vi "Parse Sonar Data.vi"(1 "Sonar Values String":string) -> (0 "Sonar Data":i32[](array[numeric]))   [LabVIEW 2020, in "Advent of Code.lvlib"]
uses:
  Advent of Code.lvlib
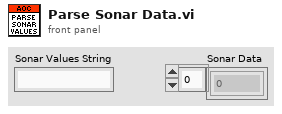
[diagram p1: front panel]
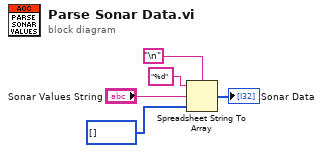
[diagram p0: block diagram]
diagram:
  n1 = Spreadsheet String To Array(delimiter (Tab)="\n", format string="%d", spreadsheet string="Sonar Values String", array type (2D Dbl)=i32[] []) -> (array=→"Sonar Data":i32[])
